vi "release entry.vi"(8 "error in (no error)":errorcluster, 10 "id":string, 11 "entry":T1) -> (0 "error out":errorcluster)   [LabVIEW 2024, in "summary manager.lvlib"]
uses:
  summary manager.lvlib
  entry type.ctl
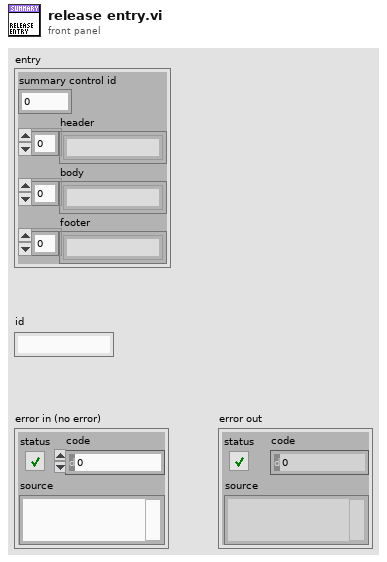
[diagram p1: front panel]
types:
  T1 = typedef "summary manager.lvlib/entry type.ctl" = cluster{"summary control id":i32, "header":string[], "body":string[], "footer":string[]}
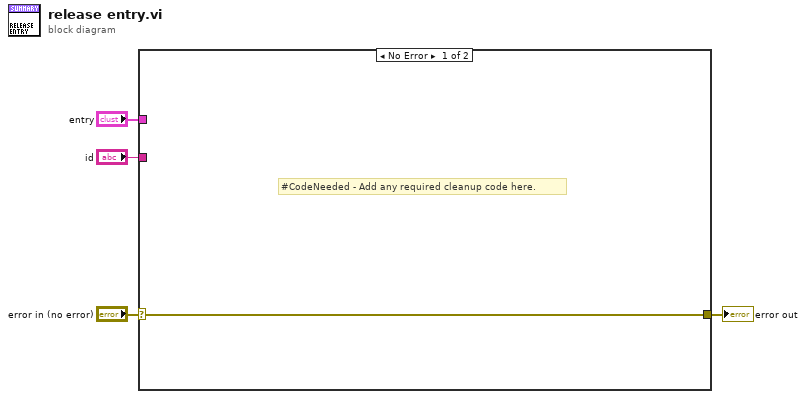
[diagram p0: block diagram]
diagram:
  n1 = case shown="No Error" "error in (no error)" {
    selector: "error in (no error)" -> [w5 w6]
    tunnel: [w5 w6] -> w3
    tunnel: "entry" -> [_ _]
    tunnel: "id" -> [_ _]
    frame No Error {
      # "#CodeNeeded - Add any required cleanup code here."
    }
    frame Error {
    }
  }
  "error out" <- w3
